vi "Music Player.vi"(10 "UI Feedback":refnum<user-event>, 11 "Command Queue":refnum<queue>) -> ()   [LabVIEW 2019, in "Sound.lvlib"]
doc: "Simple music player. Music files are played from the _Assets\\Music folder in mp3 format."
uses:
  Sound.lvlib
  Music Player Command Message.ctl
  Music Player Command.ctl
  <vilib>/sound2/lvsound2.llb/Sound Output Task ID.ctl
  Music Player State.ctl
  <vilib>/sound2/lvsound2.llb/Sampling Mode.ctl
  <vilib>/sound2/lvsound2.llb/Sound Data Format.ctl
  <vilib>/numeric/Random Number (Range) I64.vi
  <vilib>/numeric/sub_Random U32.vi
  <vilib>/sound2/lvsound2.llb/Sound Output Write (I16).vi
  _LabVIEW Audio Codecs/LabVIEW Audio Codecs.lvlib
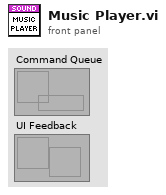
[diagram p1: front panel]
types:
  T1 = typedef "Sound.lvlib/Music Player State.ctl" = enum16{"Init Files", "Check Command", "Play", "Stop", "Shutdown"}
  T2 = typedef "Sound Output Task ID.ctl" = u32
  T3 = typedef "Sound Data Format.ctl" = cluster{"sample rate (S/s)":dbl, "number of channels":i32, "bits per sample":i32}
  T4 = typedef "Sound.lvlib/Music Player Command Message.ctl" = cluster{"Command":T5, "Data":variant}
  T5 = typedef "Sound.lvlib/Music Player Command.ctl" = enum16{"Enable", "Play", "Play Random", "Stop", "Shutdown"}
  T6 = typedef "Sampling Mode.ctl" = i32
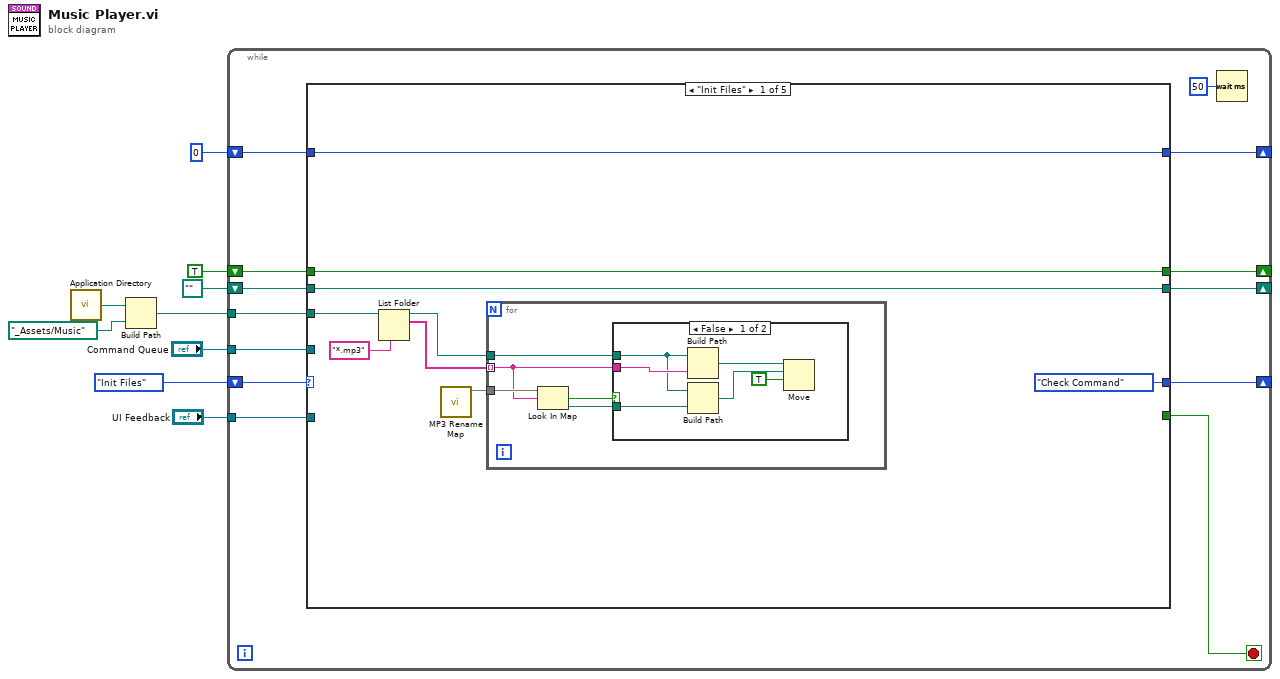
[diagram p0: block diagram]
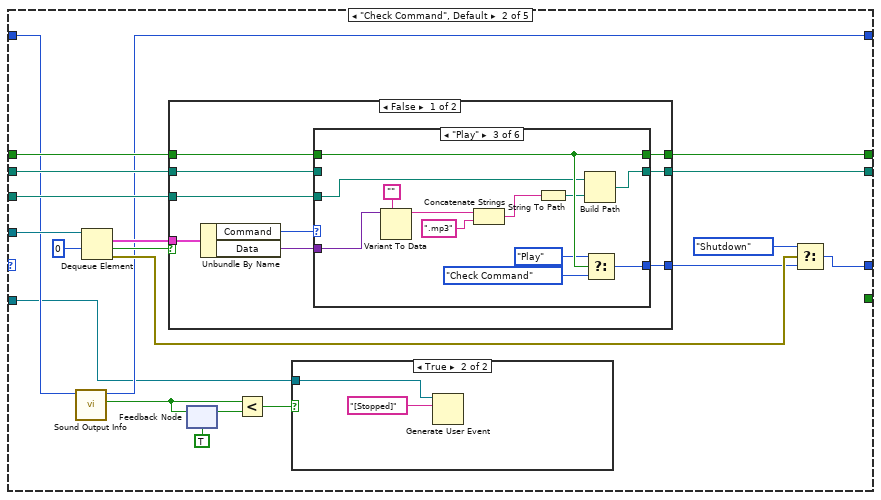
[diagram p3: hidden frame]
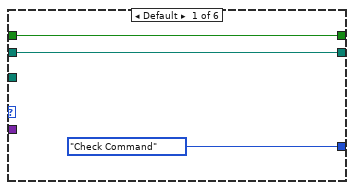
[diagram p5: hidden frame]
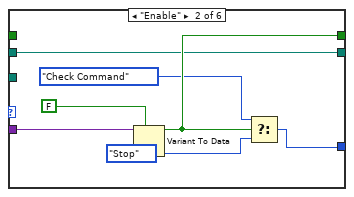
[diagram p6: hidden frame]
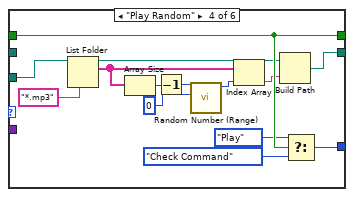
[diagram p7: hidden frame]
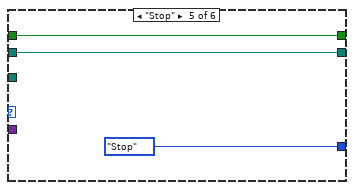
[diagram p8: hidden frame]
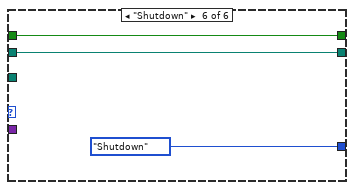
[diagram p9: hidden frame]
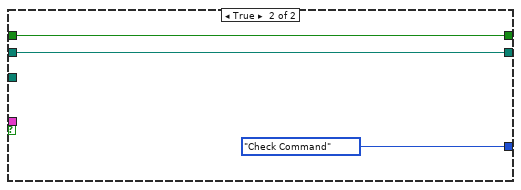
[diagram p10: hidden frame]
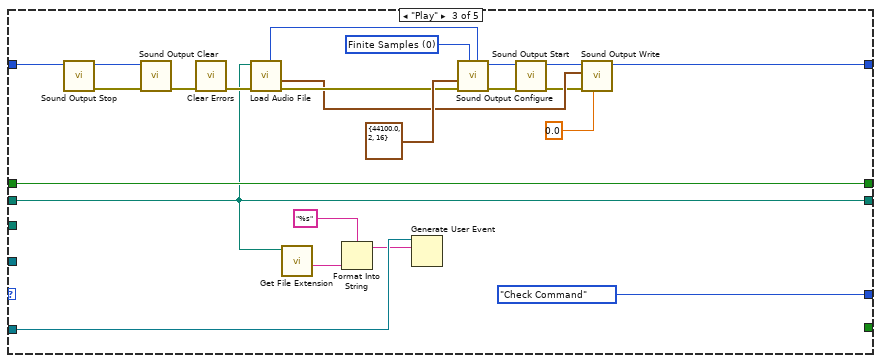
[diagram p11: hidden frame]
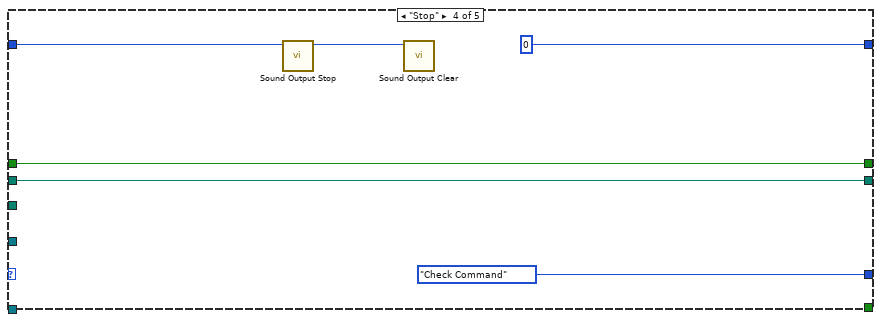
[diagram p12: hidden frame]
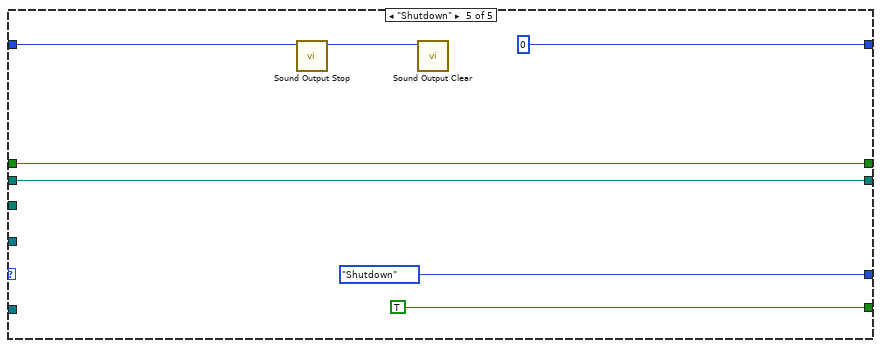
[diagram p13: hidden frame]
diagram:
  n1 = call <vilib>:"Application Directory.vi"() -> ("Application Directory"=w4:path)
  n2 = Build Path(base path=w4, name or relative path=path "_Assets/Music" ("path")) -> (appended path=w2:path)
  n3 = while {
    shift-right: [w22] -> _
    shift-left: T2 0 ("task ID out") -> [w21]
    shift-right: [w19] -> _
    shift-left: Music_Player_State."Init Files" -> [w20]
    tunnel: "Command Queue" -> [w17]
    shift-right: [w16] -> _
    shift-left: TRUE -> [w15]
    shift-right: [w14] -> _
    shift-left: path "" -> [w13]
    tunnel: w2 -> [w11]
    tunnel: "UI Feedback" -> [w10]
    stop <- w18 stop-if-true
    n4 = case shown="\"Init Files\"" w20 {
      tunnel: [w31 w45 w130 T2 0 ("task ID out") T2 0 ("task ID out")] -> w22
      tunnel: w21 -> [w31 w49 w127 w146 w148]
      tunnel: [Music_Player_State."Check Command" ("f") w52 Music_Player_State."Check Command" Music_Player_State."Check Command" ("f") Music_Player_State."Shutdown" ("f")] -> w19
      tunnel: [_ _ _ _ TRUE] -> w18
      tunnel: w17 -> [_ w62 _ _ _]
      tunnel: [w30 w58 w123 w142 w151] -> w16
      tunnel: w15 -> [w30 w57 w123 w142 w151]
      tunnel: [w29 w56 w120 w141 w150] -> w14
      tunnel: w13 -> [w29 w55 w120 w141 w150]
      tunnel: w11 -> [w26 w50 _ _ _]
      tunnel: w10 -> [_ w43 w122 _ _]
      frame "Init Files" {
        n5 = List Folder(path=w26, pattern="*.mp3") -> (path out=w23:path, filenames=w25:string[])  [unwired: 2 in, 2 out]
        n6 = call "MP3 Rename Map.vi"() -> ("MP3 Rename Map"=w24:map{string, path})  [unwired: 11 in]
        n7 = for {
          tunnel: w25 -> [w34] mode=indexing
          tunnel: w24 -> [w36]
          tunnel: w23 -> [w32]
          n8 = Look In Map(map=w36, key=w34) -> (key not found?=w35:bool, value=w33:path)  [unwired: 1 in]
          n9 = case shown="False" w35 {
            tunnel: w34 -> [w42 _]
            tunnel: w33 -> [w39 _]
            tunnel: w32 -> [w40 _]
            frame False {
              n10 = Build Path(base path=w40, name or relative path=w42) -> (appended path=w41:path)
              n11 = Build Path(base path=w40, name or relative path=w39) -> (appended path=w38:path)
              n12 = Move(source path=w41, 9:TRUE ("overwrite (F)"), 10:w38) -> ()  [unwired: 2 in, 3 out]
            }
            frame True {
            }
          }
        }
      }
      frame "Check Command", Default {
        n13 = call <vilib>:"Sound Output Info.vi"("task ID"=w49) -> ("is playing?"=w47:bool, "task ID out"=w45:T2)  [unwired: 7 in, 2 out]
        n14 = Dequeue Element(queue=w62, timeout in ms (-1)=0) -> (element=w60:T4, timed out?=w59:bool, error out=w54:errorcluster)  [unwired: 1 in, 1 out]
        n15 = case shown="False" w59 {
          tunnel: w60 -> [w73 _]
          tunnel: [w68 Music_Player_State."Check Command"] -> w53
          tunnel: [w70 w116] -> w58
          tunnel: w57 -> [w69 w116]
          tunnel: [w67 w115] -> w56
          tunnel: w55 -> [w66 w115]
          tunnel: w50 -> [w65 _]
          frame False {
            n16 = Unbundle By Name(w73) -> ("Command"=w72:T5, "Data"=w71:variant)
            n17 = case shown="\"Play\"" w72 {
              tunnel: w71 -> [_ w83 w91 _ _ _]
              tunnel: [w76 w81 w95 w108 w111 w113] -> w70
              tunnel: w69 -> [w76 _ w95 w108 w111 w113]
              tunnel: [Music_Player_State."Check Command" w80 w94 w107 Music_Player_State."Stop" ("f") Music_Player_State."Shutdown" ("f")] -> w68
              tunnel: [w74 w77 w86 w104 w110 w112] -> w67
              tunnel: w66 -> [w74 w77 _ _ w110 w112]
              tunnel: w65 -> [_ _ w85 w103 _ _]
              frame Default {
              }
              frame "Enable" {
                n18 = Variant To Data(type=FALSE, Variant=w83) -> (data=w81:bool)  [unwired: 1 in, 1 out]
                n19 = Select(t=Music_Player_State."Check Command", s=w81, f=Music_Player_State."Stop") -> (s? t:f=w80:T1)
              }
              frame "Play" {
                n20 = Variant To Data(type="", Variant=w91) -> (data=w89:string)  [unwired: 1 in, 1 out]
                n21 = Concatenate Strings(w89, ".mp3" ("string")) -> (w87:string)
                n22 = String To Path(string=w87) -> (path=w84:path)
                n23 = Build Path(base path=w85, name or relative path=w84) -> (appended path=w86:path)
                n24 = Select(t=Music_Player_State."Play", s=w95, f=Music_Player_State."Check Command") -> (s? t:f=w94:T1)
              }
              frame "Play Random" {
                n25 = List Folder(path=w103, pattern="*.mp3") -> (filenames=w100:string[])  [unwired: 2 in, 3 out]
                n26 = Array Size(array=w100) -> (size(s)=w99:i32)
                n27 = Decrement(x=w99) -> (x-1=w96:i32)
                n28 = call-poly <vilib>:"Random Number (Range).vi"("lower bound (-100)"=i64 0, "upper bound (100)"=w96) -> ("number"=w97:i64)  [unwired: 9 in]
                n29 = Index Array(array=w100, index=w97) -> (element=w101:string)
                n30 = Build Path(base path=w103, name or relative path=w101) -> (appended path=w104:path)
                n31 = Select(t=Music_Player_State."Play", s=w108, f=Music_Player_State."Check Command") -> (s? t:f=w107:T1)
              }
              frame "Stop" {
              }
              frame "Shutdown" {
              }
            }
          }
          frame True {
          }
        }
        n32 = feedback-in #1(w47) -> ()
        n33 = feedback #1(TRUE ("is playing?")) -> (w46:bool)
        n34 = Less?(x=w47, y=w46) -> (x < y?=w44:bool)
        n35 = case shown="True" w44 {
          tunnel: w43 -> [_ w64]
          frame False {
          }
          frame True {
            n36 = Generate User Event(user event=w64, event data cluster="[Stopped]" ("event data")) -> ()  [unwired: 2 in, 2 out]
          }
        }
        n37 = Select(t=Music_Player_State."Shutdown", s=w54, f=w53) -> (s? t:f=w52:T1)
      }
      frame "Play" {
        w140 = T6 0 items=["Finite Samples", "Continuous Samples"] ("sample mode")
        n38 = call <vilib>:"Sound Output Stop.vi"("task ID"=w127) -> ("error out"=w126:errorcluster, "task ID out"=w128:T2)  [unwired: 9 in]
        n39 = call <vilib>:"Sound Output Clear.vi"("error in (no error)"=w126, "task ID"=w128) -> ("error out"=w125:errorcluster)  [unwired: 9 in]
        n40 = call <vilib>:"Clear Errors.vi"("error in (no error)"=w125) -> ("error out"=w124:errorcluster)  [unwired: 5 in, 1 out]
        n41 = call "Load Audio File.vi"("error in (no error)"=w124, "Path"=w120) -> ("error out"=w137:errorcluster, "Data"=w134:waveform(i16)[], "Length (Samples)"=w138:u64)  [unwired: 5 in, 2 out]
        n42 = call <vilib>:"Get File Extension.vi"("file"=w120) -> ("filename without extension"=w119:string)  [unwired: 6 in, 4 out]
        n43 = Format Into String(format string="%s" ("event data"), w119) -> (resulting string=w118:string)  [unwired: 2 in, 1 out]
        n44 = Generate User Event(user event=w122, event data cluster=w118) -> ()  [unwired: 2 in, 2 out]
        n45 = call <vilib>:"Sound Output Configure.vi"("number of samples/ch"=w138, "sample mode"=w140, "error in (no error)"=w137, "sound format"=T3 {"sample rate (S/s)"=44100.0, "number of channels"=2, "bits per sample"=16}) -> ("error out"=w135:errorcluster, "task ID"=w136:T2)  [unwired: 6 in]
        n46 = call <vilib>:"Sound Output Start.vi"("error in (no error)"=w135, "task ID"=w136) -> ("error out"=w133:errorcluster, "task ID out"=w132:T2)  [unwired: 8 in]
        n47 = call-poly <vilib>:"Sound Output Write.vi"("timeout (sec)"=0.0, "error in (no error)"=w133, "data"=w134, "task ID"=w132) -> ("task ID out"=w130:T2)  [unwired: 6 in, 1 out]
      }
      frame "Stop" {
        n48 = call <vilib>:"Sound Output Stop.vi"("task ID"=w146) -> ("task ID out"=w145:T2)  [unwired: 9 in, 1 out]
        n49 = call <vilib>:"Sound Output Clear.vi"("task ID"=w145) -> ()  [unwired: 10 in, 1 out]
      }
      frame "Shutdown" {
        n50 = call <vilib>:"Sound Output Stop.vi"("task ID"=w148) -> ("task ID out"=w149:T2)  [unwired: 9 in, 1 out]
        n51 = call <vilib>:"Sound Output Clear.vi"("task ID"=w149) -> ()  [unwired: 10 in, 1 out]
      }
    }
    n52 = Wait (ms)(milliseconds to wait=u32 50) -> ()  [unwired: 1 out]
  }
